vi "I2C Close.vi"(7 "I2C Channel":u8, 8 "Error In":errorcluster, 11 "LINX Device Config":T1) -> (0 "Error Out":errorcluster, 3 "LINX Device Config":T1)   [LabVIEW 2011, in "LVH-LINX.lvlib" / "Device.lvlib"]
doc: "Close the specified I2C channel."
uses:
  Device.lvlib
  Type Defs/LINX Device Config.ctl
  Type Defs/Interface.ctl
  Type Defs/TCP Config.ctl
  Type Defs/Device Family.ctl
  Type Defs/Error Type.ctl
  LVH-LINX.lvlib
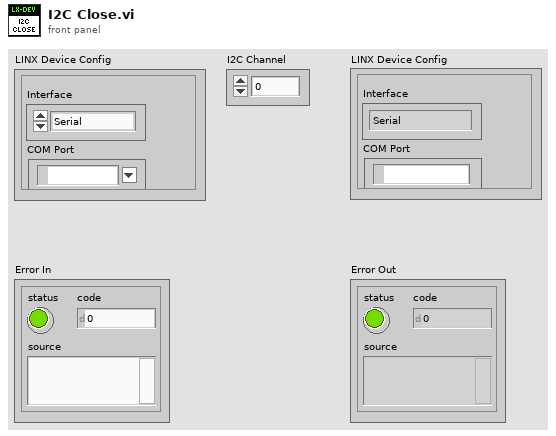
[diagram p1: front panel]
types:
  T1 = typedef "LVH-LINX.lvlib/Device.lvlib/LINX Device Config.ctl" = cluster{"Interface":T2, "COM Port":refnum<visa-resource-name>, "TCP Configuration":T3, "Device Family":T4, "Device ID":u8, "Device Name":string, "TCP Ref":refnum<k5>}
  T2 = typedef "LVH-LINX.lvlib/Interface.ctl" = enum16{"Serial", "TCP"}
  T3 = typedef "LVH-LINX.lvlib/Device.lvlib/TCP Config.ctl" = cluster{"IP Address":string, "Port":u16}
  T4 = typedef "LVH-LINX.lvlib/Device Family.ctl" = enum8{"National Instruments", "Digilent", "Arduino"}
  T5 = typedef "LVH-LINX.lvlib/Error Type.ctl" = enum16{"Unknown", "Timeout", "Corrupt Return Packet", "Unable To Connect", "Command Not Supported", "Channel DNE", "Invalid COM Config"}
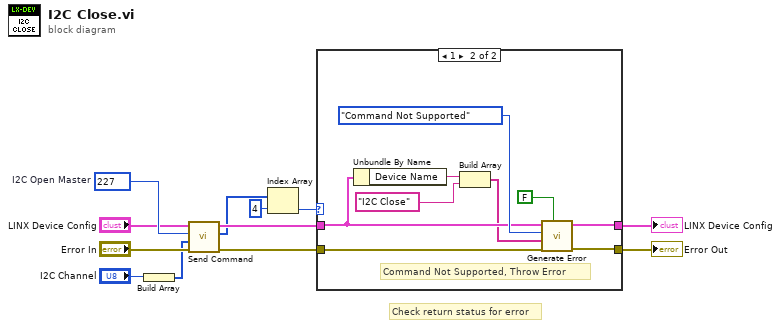
[diagram p0: block diagram]
diagram:
  w11 = u16 227  # I2C Open Master
  # "Check return status for error"
  n1 = Build Array("I2C Channel") -> (w1:u8[])
  n2 = call "Send Command.vi"("Error In"="Error In", "ARGS"=w1, "CMD"=w11, "LINX Device Config"="LINX Device Config") -> ("Error Out"=w4:errorcluster, "Response"=w3:u8[], "LINX Device Config"=w6:T1)  [unwired: 4 in, 1 out]
  n3 = Index Array(array=w3, index=4) -> (element=w8:u8)
  n4 = case shown="1" w8 {
    tunnel: [w14 w21] -> w7
    tunnel: w6 -> [w14 w17]
    tunnel: [w13 w22] -> w5
    tunnel: w4 -> [w13 w23]
    frame 0, Default {
      # "Status OK, No Data To Process"
    }
    frame 1 {
      # "Command Not Supported, Throw Error"
      n5 = Unbundle By Name(w17) -> ("Device Name"=w19:string)
      n6 = Build Array(w19, "I2C Close") -> (w16:string[])
      n7 = call "Generate Error.vi"("Is Warning? (False)"=FALSE, "Error In"=w23, "Arguments"=w16, "Error Type"=Error_Type."Command Not Supported", "LINX Device Config"=w17) -> ("Error Out"=w22:errorcluster, "LINX Device Config"=w21:T1)  [unwired: 5 in]
    }
  }
  "Error Out" <- w5
  "LINX Device Config" <- w7
